vi "Re-Origin.vi"(9 "Transition":cluster{"X Delta":dbl, "Y Delta":dbl}, 10 "Y":dbl[](array[numeric]), 11 "X":dbl[](array[numeric])) -> (2 "Normalized Y":dbl[](array[numeric]), 3 "Normalized X":dbl[](array[numeric]))   [LabVIEW 2017]
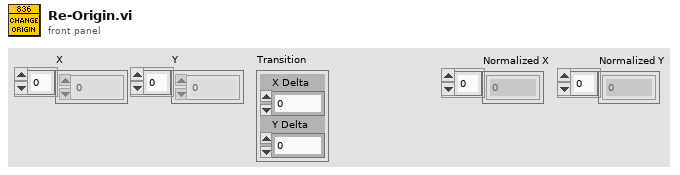
[diagram p1: front panel]
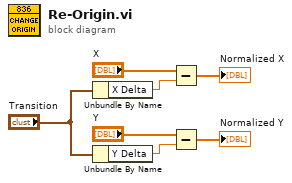
[diagram p0: block diagram]
diagram:
  n1 = Unbundle By Name("Transition") -> ("X Delta"=w7:dbl)
  n2 = Unbundle By Name("Transition") -> ("Y Delta"=w5:dbl)
  n3 = Subtract(x="X", y=w7) -> (x-y=→"Normalized X":dbl[])
  n4 = Subtract(x="Y", y=w5) -> (x-y=→"Normalized Y":dbl[])
